vi "LV to ITX XY2 AutoPlot.vi"(0 "filename":string="filename", 1 "path":path=path "C:/", 5 "Notes":string, 7 "Data":cluster{"Y  Array":dbl[]}[](array[cluster]), 11 "wavenames (.Vx, etc)":string[](array[string])=["time", "x", "y", "z"], 12 "X,Y Labels":string[](array[string])=["x label", "y label"], 13 "X,Y Log":i32[](array[numeric]), 14 "input command string":string="Display/R '#wave#'\nAppendToGraph '#wave#'\nLabel bottom \"#labelX#\"\nLabel left \"#labelY#\"\nModifyGraph rgb('#wave#')=(#r#,#g#,#b#)\n\\\\s('#wave#') #label#\nModifyGraph mirror(bottom)=1\nModifyGraph width=216\nModifyGraph height={Aspect,0.6}\nModifyGraph Log(bottom)=#bottomlog#\nModifyGraph Log(left)=#leftlog#") -> (4 "file":path)   [LabVIEW 2016, in "LVtoITX.lvclass"]
doc: "Write data to ITX file. This AutoPlot VI adds commands to automatically create a graph in Igor to quickly view your data.\n\n-- path: base path to save data\n-- filename: base filename\n-- Notes: add any notes here to help you remember what experiment you did\n-- Data: Cluster array\n It is recommended that you make the first cluster an array of timestamps\n-- wavenames: Give each data array a unique name such as \"time, bias, current,...\"zz\n-- X,Y Labels: For plotting in Igor. Can be ignored.\n-- X,Y Log: Do you wan to show X or Y on Log scale in Igor?"
uses:
  LVtoITX.lvclass
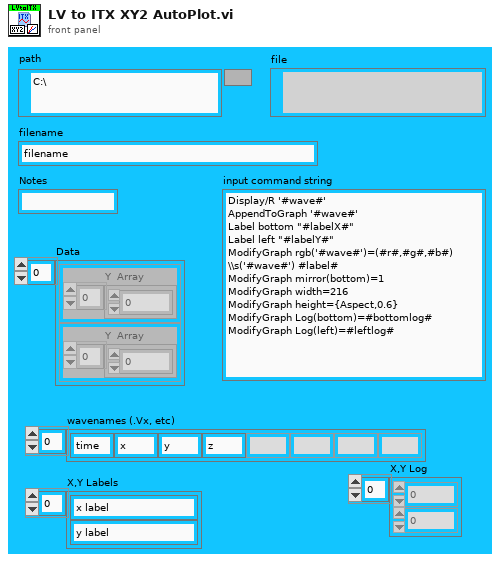
[diagram p1: front panel]
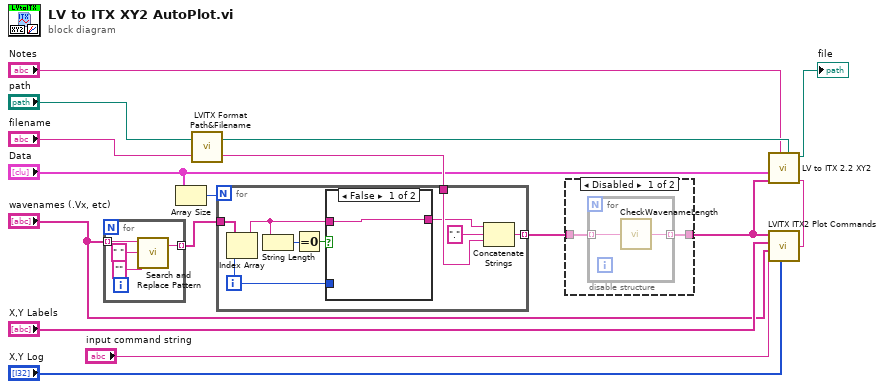
[diagram p0: block diagram]
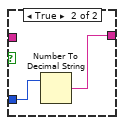
[diagram p3: hidden frame]
diagram:
  n1 = for {
    tunnel: "wavenames (.Vx, etc)" -> [w18] mode=indexing
    tunnel: [w17] -> w5 mode=indexing
    n2 = call <vilib>:"Search and Replace Pattern.vi"("string"=w18, "regular expression (\"\")"=" " ("regular expression (\"\")"), "replace string (\"\")"="" ("replace string (\"\")")) -> ("result string"=w17:string)  [unwired: 2 in, 1 out]
  }
  n3 = Array Size(array="Data") -> (size(s)=w15:i32)
  n4 = call "LVITX Format Path&Filename.vi"("filename"="filename", "path"="path") -> ("file name without extension"=w14:string, "dup file"=w12:path)
  n5 = for {
    N: w15 -> [_]
    tunnel: w5 -> [w24]
    tunnel: w14 -> [w22]
    tunnel: [w29] -> w3 mode=indexing
    i -> [w25]
    n6 = Index Array(array=w24, index=w25) -> (element=w23:string)
    n7 = String Length(string=w23) -> (length=w26:i32)
    n8 = Equal To 0?(x=w26) -> (x = 0?=w27:bool)
    n9 = case shown="False" w27 {
      tunnel: w25 -> [_ w31]
      tunnel: [w30 w32] -> w21
      tunnel: w23 -> [w30 _]
      frame False {
      }
      frame True {
        n10 = Number To Decimal String(number=w31) -> (decimal integer string=w32:string)  [unwired: 1 out]
      }
    }
    n11 = Concatenate Strings(w21, "." ("string"), w22) -> (w29:string)
  }
  n12 = disable-structure shown="Disabled" {
    disable-tunnel: w3 -> [w34 w37]
    disable-tunnel: [w33 w37] -> w2
    frame Disabled {
      n13 = for {
        tunnel: w34 -> [w36] mode=indexing
        tunnel: [w35] -> w33 mode=indexing
        n14 = call "CheckWavenameLength.vi"("wavename"=w36) -> ("wavename"=w35:string)
      }
    }
    frame Enabled {
    }
  }
  n15 = call "LVITX ITX2 Plot Commands.vi"("X,Y Log"="X,Y Log", "input string"="input command string", "Plot labels"="wavenames (.Vx, etc)", "X,Y Labels"="X,Y Labels", "wavenames"=w2) -> ("result string"=w4:string)  [unwired: 1 in]
  n16 = call "LV to ITX 2.2 XY2.vi"("Commands"=w4, "filename"=w12, "Notes"="Notes", "wavenames"=w2, "array of clusters"="Data") -> ("file"=→"file":path)  [unwired: 6 in]
